vi "WriteHEWHData.vi"() -> ()   [LabVIEW 2009]
uses:
  <vilib>/Utility/file.llb/Write To Spreadsheet File (string).vi
  EquipReferences.ctl
panel:
  in  "Include Header?":bool
  out "error out":errorcluster
  in  "Equipment":T1={"COM Port"="COM1", "MW100"="MW100", "AG34970"="A-34972A", "WT500"="WT500"}
  in  "error in (no error)":errorcluster
  in  "Semiphore":T2
  out "Output Data":string[][](array[string])
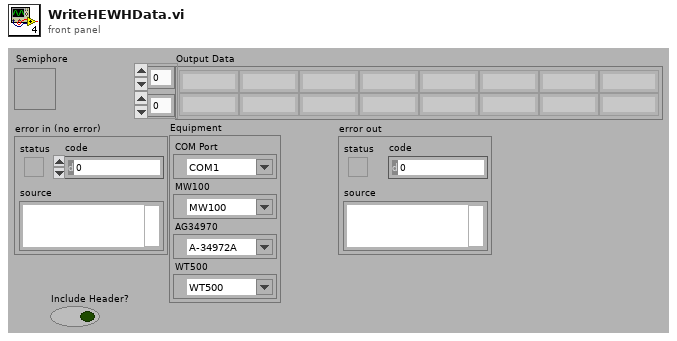
[diagram p1: front panel]
types:
  T1 = typedef "EquipReferences.ctl" = cluster{"COM Port":refnum<visa-resource-name>, "MW100":refnum<visa-resource-name>, "AG34970":refnum<visa-resource-name>, "WT500":refnum<visa-resource-name>}
  T2 = typedef "Semaphore RefNum" = refnum<k1>
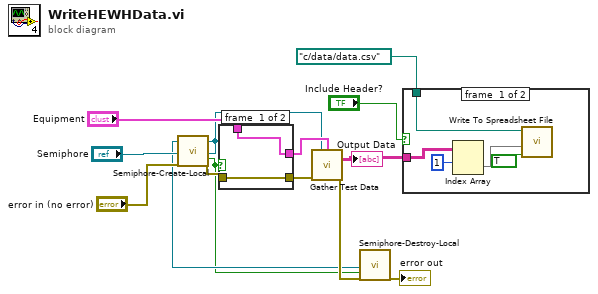
[diagram p0: block diagram]
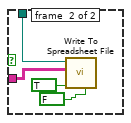
[diagram p2: hidden frame]
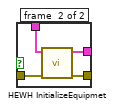
[diagram p3: hidden frame]
diagram:
  n1 = call "Semiphore-Create-Local.vi"("Semiphore"="Semiphore", "error in (no error)"="error in (no error)") -> ("semaphore"=w6:T2, "Local?"=w5:bool, "error out"=w13:errorcluster)  [unwired: 15 in]
  n2 = case shown="True" w5 {
    tunnel: w13 -> [w14 w19]
    tunnel: "Equipment" -> [w15 w18]
    tunnel: [w15 w17] -> w9
    tunnel: [w14 w16] -> w8
    frame #0 {
    }
    frame #1 {
      n3 = call "HEWH InitializeEquipmet.vi"("Error In"=w19, "Equipment"=w18) -> ("Error Out"=w16:errorcluster, "Equipment Out"=w17:T1)  [unwired: 8 in]
    }
  }
  n4 = call "Gather Test Data.vi"("Semiphore"=w6, "Equipment"=w9, "error in (no error)"=w8) -> ("Output Data"=w3:string[][], "error out"=w7:errorcluster)  [unwired: 11 in]
  "Output Data" <- w3
  n5 = call "Semiphore-Destroy-Local.vi"("Semiphore"=w6, "Local?"=w5, "error in (no error)"=w7) -> ("error out"=→"error out":errorcluster)  [unwired: 16 in]
  n6 = case shown="False" "Include Header?" {
    tunnel: w3 -> [w24 w26]
    tunnel: path "c:/data/data.csv" ("file path (dialog if empty)") -> [w20 w25]
    frame #0 {
      n7 = Index Array(array=w24, index (row)=1) -> (element=w22:string[])  [unwired: 1 in]
      n8 = call-poly <vilib>:"Write To Spreadsheet File.vi"("append to file? (new file:F)"=TRUE, "1D data"=w22, "file path (dialog if empty)"=w20) -> ()  [unwired: 5 in, 1 out]
    }
    frame #1 {
      n9 = call-poly <vilib>:"Write To Spreadsheet File.vi"("transpose? (no:F)"=FALSE, "append to file? (new file:F)"=TRUE, "2D data"=w26, "file path (dialog if empty)"=w25) -> ()  [unwired: 4 in, 1 out]
    }
  }
